vi "Lock-in save info (SubVI).vi"(8 "error in (no error)":errorcluster, 11 "Instrument parameters in":T1) -> (0 "error out":errorcluster, 2 "Array":string[][](array[string]), 3 "Instrument parameters out":T1)   [LabVIEW 2025]
uses:
  TYPE DEFS/S2DS_Instrument parameters.ctl
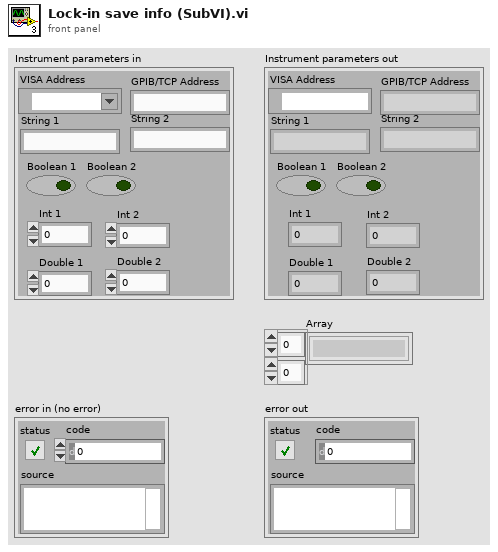
[diagram p1: front panel]
types:
  T1 = typedef "S2DS_Instrument parameters.ctl" = cluster{"VISA Address":refnum<visa-resource-name>, "GPIB/TCP Address":string, "String 1":string, "String 2":string, "Boolean 1":bool, "Boolean 2":bool, "Int 1":i32, "Int 2":i32, "Double 1":dbl, "Double 2":dbl}
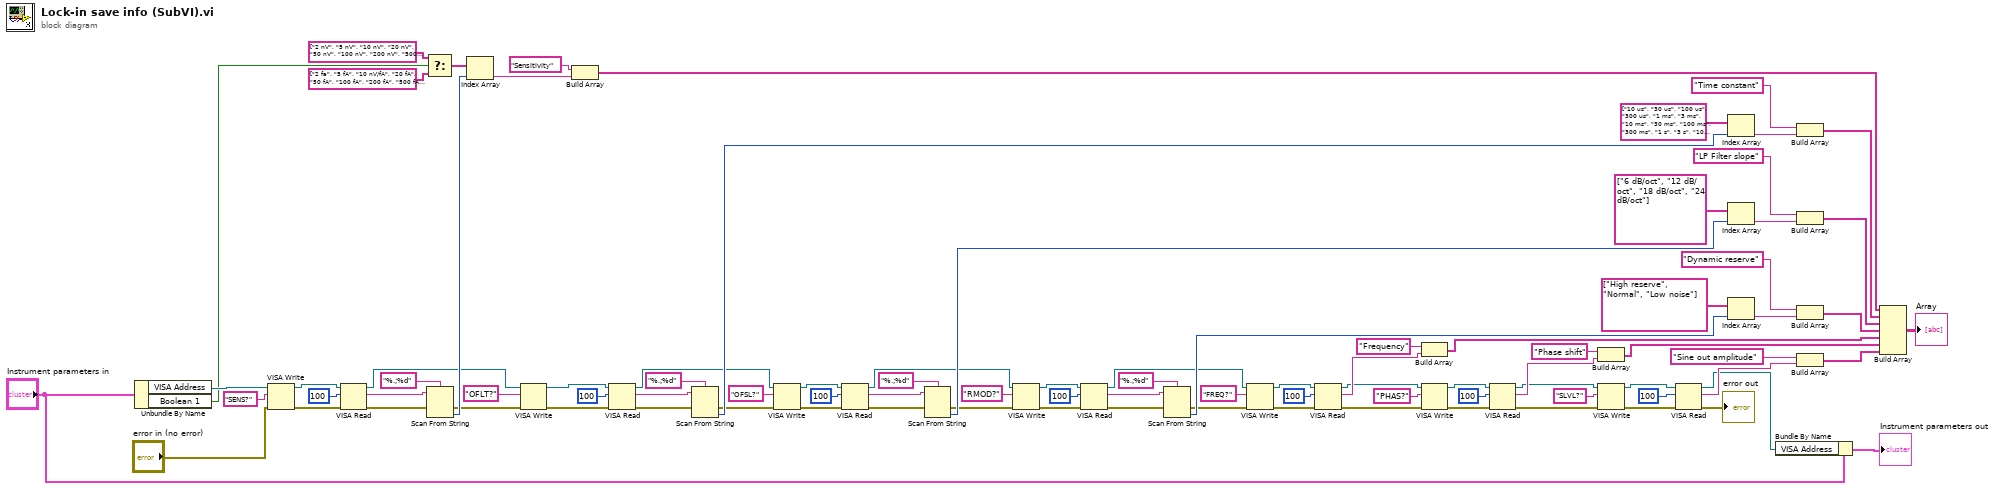
[diagram p0: block diagram]
diagram:
  n1 = Unbundle By Name("Instrument parameters in") -> ("VISA Address"=w89:refnum<visa-resource-name>, "Boolean 1"=w76:bool)
  n2 = VISA Write(VISA resource name=w89, write buffer="SENS?", error in (no error)="error in (no error)") -> (VISA resource name out=w88:refnum<visa-resource-name>, error out=w90:errorcluster)  [unwired: 1 out]
  n3 = VISA Read(VISA resource name=w88, byte count=u32 100, error in (no error)=w90) -> (VISA resource name out=w66:refnum<visa-resource-name>, read buffer=w80:string, error out=w79:errorcluster)  [unwired: 1 out]
  n4 = Select(t=string[] ["2 nV", "5 nV", "10 nV", "20 nV", "50 nV", "100 nV", "200 nV", "500 nV", "1 uV", "2 uV", "5 uV", "10 uV", "20 uV", "50 uV", "100 uV", "200 uV", "500 uV", "1 mV", "2 mV", "5 mV", "10 mV", "20 mV", "50 mV", "100 mV", "200 mV", "500 mV", "1 V", "Error"], s=w76, f=string[] ["2 fa", "5 fA", "10 nV/fA", "20 fA", "50 fA", "100 fA", "200 fA", "500 fA", "1 pA", "2 pA", "5 pA", "10 pA", "20 pA", "50 pA", "100 pA", "200 pA", "500 pA", "1 nA", "2 nA", "5 nA", "10 nA", "20 nA", "50 nA", "100 nA", "200 nA", "500 nA", "1 uA", "Error"]) -> (s? t:f=w75:string[])
  n5 = Scan From String(format string="%.;%d", input string=w80, error in=w79) -> (error out=w67:errorcluster, output 1=w81:i32)  [unwired: 2 in, 2 out]
  n6 = Index Array(array=w75, index=w81) -> (element=w74:string)
  n7 = VISA Write(VISA resource name=w66, write buffer="OFLT?", error in (no error)=w67) -> (VISA resource name out=w71:refnum<visa-resource-name>, error out=w72:errorcluster)  [unwired: 1 out]
  n8 = Build Array("Sensitivity", w74) -> (w85:string[])
  n9 = VISA Read(VISA resource name=w71, byte count=u32 100, error in (no error)=w72) -> (VISA resource name out=w52:refnum<visa-resource-name>, read buffer=w69:string, error out=w68:errorcluster)  [unwired: 1 out]
  n10 = Scan From String(format string="%.;%d", input string=w69, error in=w68) -> (error out=w53:errorcluster, output 1=w64:i32)  [unwired: 2 in, 2 out]
  n11 = VISA Write(VISA resource name=w52, write buffer="OFSL?", error in (no error)=w53) -> (VISA resource name out=w57:refnum<visa-resource-name>, error out=w58:errorcluster)  [unwired: 1 out]
  n12 = VISA Read(VISA resource name=w57, byte count=u32 100, error in (no error)=w58) -> (VISA resource name out=w38:refnum<visa-resource-name>, read buffer=w55:string, error out=w54:errorcluster)  [unwired: 1 out]
  n13 = Scan From String(format string="%.;%d", input string=w55, error in=w54) -> (error out=w39:errorcluster, output 1=w50:i32)  [unwired: 2 in, 2 out]
  n14 = VISA Write(VISA resource name=w38, write buffer="RMOD?", error in (no error)=w39) -> (VISA resource name out=w43:refnum<visa-resource-name>, error out=w44:errorcluster)  [unwired: 1 out]
  n15 = VISA Read(VISA resource name=w43, byte count=u32 100, error in (no error)=w44) -> (VISA resource name out=w27:refnum<visa-resource-name>, read buffer=w41:string, error out=w40:errorcluster)  [unwired: 1 out]
  n16 = Scan From String(format string="%.;%d", input string=w41, error in=w40) -> (error out=w28:errorcluster, output 1=w36:i32)  [unwired: 2 in, 2 out]
  n17 = VISA Write(VISA resource name=w27, write buffer="FREQ?", error in (no error)=w28) -> (VISA resource name out=w26:refnum<visa-resource-name>, error out=w30:errorcluster)  [unwired: 1 out]
  n18 = VISA Read(VISA resource name=w26, byte count=u32 100, error in (no error)=w30) -> (VISA resource name out=w18:refnum<visa-resource-name>, read buffer=w25:string, error out=w17:errorcluster)  [unwired: 1 out]
  n19 = Build Array("Frequency" ("element"), w25) -> (w23:string[])
  n20 = VISA Write(VISA resource name=w18, write buffer="PHAS?", error in (no error)=w17) -> (VISA resource name out=w16:refnum<visa-resource-name>, error out=w21:errorcluster)  [unwired: 1 out]
  n21 = VISA Read(VISA resource name=w16, byte count=u32 100, error in (no error)=w21) -> (VISA resource name out=w7:refnum<visa-resource-name>, read buffer=w19:string, error out=w6:errorcluster)  [unwired: 1 out]
  n22 = Build Array("Phase shift" ("element"), w19) -> (w14:string[])
  n23 = VISA Write(VISA resource name=w7, write buffer="SLVL?", error in (no error)=w6) -> (VISA resource name out=w9:refnum<visa-resource-name>, error out=w12:errorcluster)  [unwired: 1 out]
  n24 = VISA Read(VISA resource name=w9, byte count=u32 100, error in (no error)=w12) -> (VISA resource name out=w1:refnum<visa-resource-name>, read buffer=w10:string, error out=→"error out":errorcluster)  [unwired: 1 out]
  n25 = Index Array(array=string[] ["10 us", "30 us", "100 us", "300 us", "1 ms", "3 ms", "10 ms", "30 ms", "100 ms", "300 ms", "1 s", "3 s", "10 s", "30 s", "100 s", "300 s", "1 ks", "3 ks", "10 ks", "30 ks", "Error"], index=w64) -> (element=w62:string)
  n26 = Index Array(array=string[] ["6 dB/oct", "12 dB/oct", "18 dB/oct", "24 dB/oct"], index=w50) -> (element=w48:string)
  n27 = Index Array(array=string[] ["High reserve", "Normal", "Low noise"], index=w36) -> (element=w34:string)
  n28 = Bundle By Name(cluster="Instrument parameters in", "VISA Address"=w1) -> (→"Instrument parameters out":T1)
  n29 = Build Array("Time constant" ("element"), w62) -> (w60:string[])
  n30 = Build Array("LP Filter slope" ("element"), w48) -> (w46:string[])
  n31 = Build Array("Dynamic reserve" ("element"), w34) -> (w32:string[])
  n32 = Build Array("Sine out amplitude" ("element"), w10) -> (w5:string[])
  n33 = Build Array(w85, w60, w46, w32, w23, w14, w5) -> (→"Array":string[][])
